vi "RPC Open App Reference.vi"(7 "Port Number (3363)":u16=3363, 8 "error in (no error)":errorcluster, 11 "Client (\"\": open server reference)":string) -> (0 "error out":errorcluster, 2 "Component Base Path":path, 3 "App Reference":refnum<vi>)   [LabVIEW 2011]
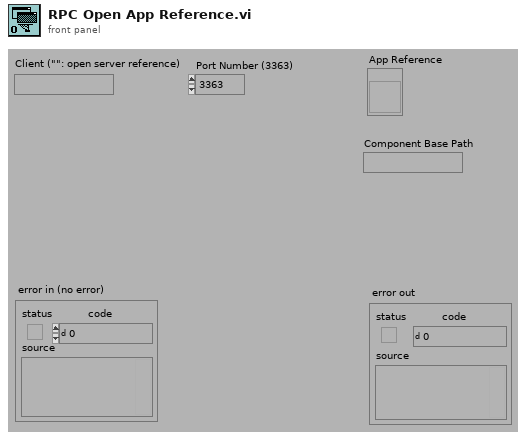
[diagram p1: front panel]
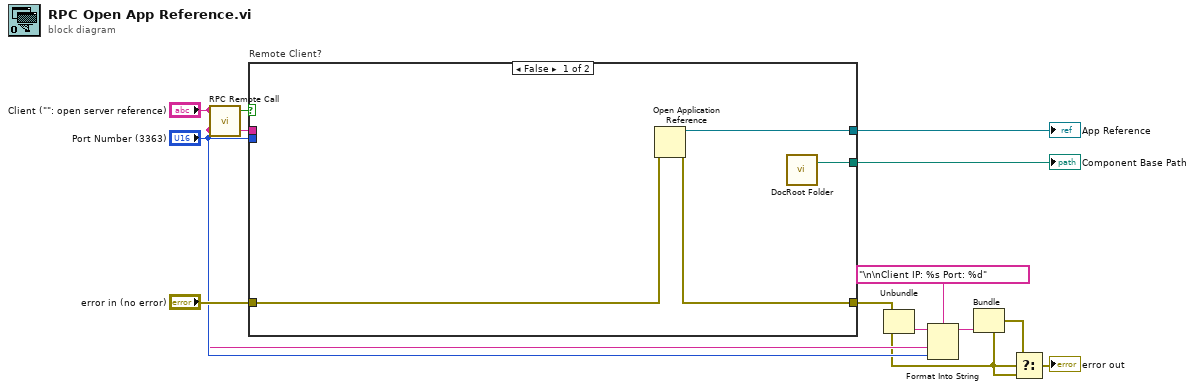
[diagram p0: block diagram]
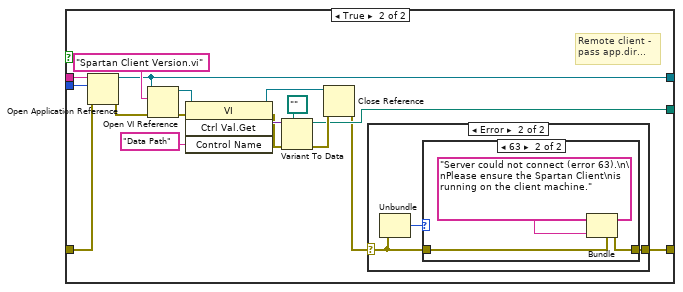
[diagram p2: hidden frame]
diagram:
  n1 = call "RPC Remote Call.vi"("IP (\"\")"="Client (\"\": open server reference)") -> ("Remote Call?"=w8:bool)  [unwired: 4 out]
  n2 = case "Remote Client?" shown="False" w8 {
    tunnel: [w15 w19] -> w3
    tunnel: [w16 w20] -> w7
    tunnel: "error in (no error)" -> [w14 w31]
    tunnel: "Port Number (3363)" -> [_ w32]
    tunnel: "Client (\"\": open server reference)" -> [_ w33]
    tunnel: [w13 w30] -> w1
    frame False {
      n3 = Open Application Reference(8:w14) -> (0:w13:errorcluster, 3:w15:refnum<vi>)  [unwired: 3 in]
      n4 = call "DocRoot Folder.vi"() -> ("DocumentRoot Folder"=w16:path)  [unwired: 3 in]
    }
    frame True {
      # "Remote client -\npass app.dir..."
      n5 = Open Application Reference(8:w31, 10:w32, 11:w33) -> (0:w18:errorcluster, 3:w19:refnum<vi>)  [unwired: 1 out]
      n6 = Open VI Reference(application reference (local)=w19, vi path="Spartan Client Version.vi" ("y"), error in (no error)=w18) -> (vi reference=w26:refnum<vi>, error out=w27:errorcluster)  [unwired: 3 out]
      n7 = invoke class="VI" method="Ctrl Val.Get"(reference=w26, error in=w27, "Control Name"="Data Path" ("y")) -> (reference out=w22:refnum<vi>, error out=w21:errorcluster, "Get Control Value Variant"=w24:variant)  [unwired: 1 in, 1 out]
      n8 = Variant To Data(error in=w21, type=path "", Variant=w24) -> (data=w20:path, error out=w25:errorcluster)
      n9 = Close Reference(reference=w22, error in (no error)=w25) -> (error out=w17:errorcluster)
      n10 = case shown="Error" w17 {
        selector: w17 -> [w34 w36]
        tunnel: [w34 w35] -> w30
        frame No Error {
        }
        frame Error {
          n11 = Unbundle(w36) -> ("code"=w37:i32)  [unwired: 2 out]
          n12 = case shown="63" w37 {
            tunnel: w36 -> [w38 w41]
            tunnel: [w38 w40] -> w35
            frame 0, Default {
            }
            frame 63 {
              n13 = Bundle(cluster=w41, "source"="Server could not connect (error 63).\n\nPlease ensure the Spartan Client\nis running on the client machine.") -> (w40:errorcluster)  [unwired: 2 out]
            }
          }
        }
      }
    }
  }
  "App Reference" <- w3
  "Component Base Path" <- w7
  n14 = Unbundle(w1) -> ("source"=w11:string)  [unwired: 2 out]
  n15 = Format Into String(format string="\n\nClient IP: %s Port: %d", initial string=w11, "Client (\"\": open server reference)", "Port Number (3363)") -> (resulting string=w12:string)  [unwired: 1 in, 1 out]
  n16 = Bundle(cluster=w1, "source"=w12) -> (w10:errorcluster)  [unwired: 2 out]
  n17 = Select(t=w10, s=w1, f=w1) -> (s? t:f=→"error out":errorcluster)
